vi "Addon.GetRef.vi"(8 "error in (no error)":errorcluster, 11 "Node Ptr":u64) -> (0 "error out":errorcluster, 2 "Addon Ref":T1 format="%.0x", 3 "Node Ptr":T1 format="%.0x")   [LabVIEW 2019, in "Diagnostics Addon System Explorer.lvlib"]
uses:
  Diagnostics Addon System Explorer.lvlib
  <vilib>/NI VeriStand/Custom Device API/Custom Device Item Ref.ctl
  <vilib>/NI VeriStand/Custom Device Tools/Custom Device Utility Library/Search Direction.ctl
  Shared/SubVIs/Constants.vi
  <vilib>/NI VeriStand/Custom Device Tools/Custom Device Utility Library/NI VeriStand - Search for Item by GUID.vi
  <vilib>/NI VeriStand/Custom Device Tools/Custom Device Utility Library/Custom Device Utility Library.lvlib
  Shared/Diagnostics Addon Shared.lvlib
  <vilib>/NI VeriStand/Custom Device API/Custom Device API.lvlib
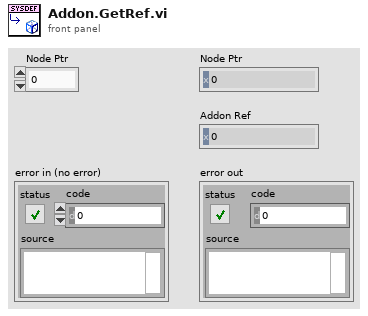
[diagram p1: front panel]
types:
  T1 = typedef "Custom Device API.lvlib/Custom Device Item Ref.ctl" = u64
  T2 = typedef "Custom Device Utility Library.lvlib/Search Direction.ctl" = enum16{"Down", "Up"}
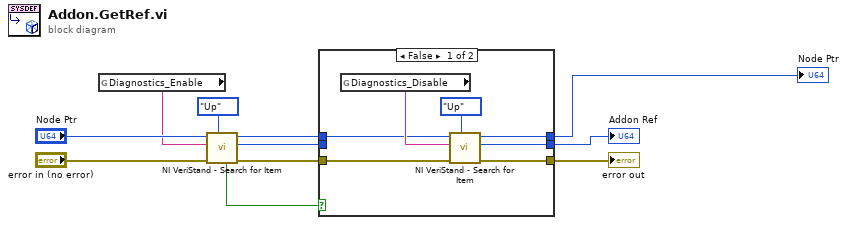
[diagram p0: block diagram]
diagram:
  n1 = global read "Constants.vi" "Diagnostics_Enable"() -> (w1:string)
  n2 = call-poly <vilib>:"NI VeriStand - Search for Item.vi"("Direction (Down)"=Search_Direction."Up", "error in"="error in (no error)", "Item GUID"=w1, "Section Ref in"="Node Ptr") -> ("error out"=w5:errorcluster, "Item Ref"=w11:T1, "Section Ref out"=w6:T1, "Found"=w10:bool)  [unwired: 4 in]
  n3 = case shown="False" w10 {
    tunnel: w5 -> [w16 w21]
    tunnel: w6 -> [w15 w20]
    tunnel: [w14 w20] -> w7
    tunnel: [w13 w19] -> w8
    tunnel: [w12 w21] -> w9
    tunnel: w11 -> [_ w19]
    frame False {
      n4 = global read "Constants.vi" "Diagnostics_Disable"() -> (w17:string)
      n5 = call-poly <vilib>:"NI VeriStand - Search for Item.vi"("Direction (Down)"=Search_Direction."Up", "error in"=w16, "Item GUID"=w17, "Section Ref in"=w15) -> ("error out"=w12:errorcluster, "Item Ref"=w13:T1, "Section Ref out"=w14:T1)  [unwired: 4 in, 1 out]
    }
    frame True {
    }
  }
  "error out" <- w9
  "Addon Ref" <- w8
  "Node Ptr" <- w7
